vi "HIOKI PW3390 Conf Measure Item sub2.vi"(1 "U or I":T1) -> (0 "U or I out":bool[][](array[boolean]))   [LabVIEW 2009]
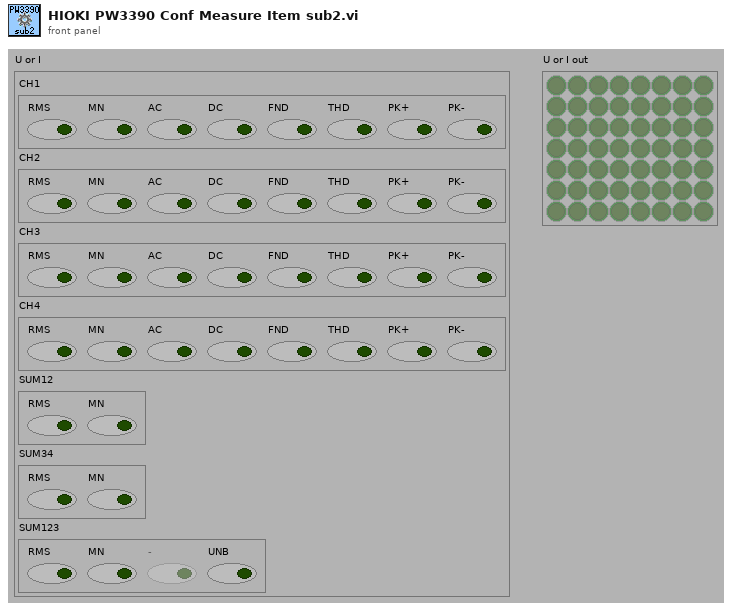
[diagram p1: front panel]
types:
  T1 = cluster{"CH1":cluster{"RMS":bool, "MN":bool, "AC":bool, "DC":bool, "FND":bool, "THD":bool, "PK+":bool, "PK-":bool}, "CH2":cluster{"RMS":bool, "MN":bool, "AC":bool, "DC":bool, "FND":bool, "THD":bool, "PK+":bool, "PK-":bool}, "CH3":cluster{"RMS":bool, "MN":bool, "AC":bool, "DC":bool, "FND":bool, "THD":bool, "PK+":bool, "PK-":bool}, "CH4":cluster{"RMS":bool, "MN":bool, "AC":bool, "DC":bool, "FND":bool, "THD":bool, "PK+":bool, "PK-":bool}, "SUM12":cluster{"RMS":bool, "MN":bool}, "SUM34":cluster{"RMS":bool, "MN":bool}, "SUM123":cluster{"RMS":bool, "MN":bool, "-":bool, "UNB":bool}}
  T2 = cluster{"RMS":bool, "MN":bool, "AC":bool, "DC":bool, "FND":bool, "THD":bool, "PK+":bool, "PK-":bool}
  T3 = cluster{"RMS":bool, "MN":bool, "-":bool, "UNB":bool}
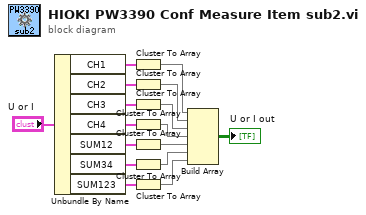
[diagram p0: block diagram]
diagram:
  n1 = Unbundle By Name("U or I") -> ("CH1"=w8:T2, "CH2"=w7:T2, "CH3"=w6:T2, "CH4"=w5:T2, "SUM12"=w4:cluster{"RMS":bool, "MN":bool}, "SUM34"=w3:cluster{"RMS":bool, "MN":bool}, "SUM123"=w2:T3)
  n2 = Cluster To Array(cluster=w8) -> (array=w10:bool[])
  n3 = Cluster To Array(cluster=w7) -> (array=w11:bool[])
  n4 = Cluster To Array(cluster=w6) -> (array=w12:bool[])
  n5 = Cluster To Array(cluster=w5) -> (array=w13:bool[])
  n6 = Cluster To Array(cluster=w4) -> (array=w14:bool[])
  n7 = Cluster To Array(cluster=w3) -> (array=w15:bool[])
  n8 = Cluster To Array(cluster=w2) -> (array=w1:bool[])
  n9 = Build Array(w10, w11, w12, w13, w14, w15, w1) -> (→"U or I out":bool[][])
